vi "Hardware-HHCmdCalPoints.vi"(0 "HH Setup In":T1[](array[typedef]) {"Skip Fire Index" max=7; "Angles"."Duration [s]" format="%#_3p"; "Frequency [Hz]" format="%#_3p"}) -> (4 "HH Setup Out":T1[](array[typedef])=[{"Mode"=enum."Off", "Digital Input"=enum."Unused", "Polarity"=FALSE, "Frequency [Hz]"=0.0, "Duty Cycle [%]"=0.0, "TDC Offset [CAD]"=0.0, "Window Start [DBTDC]"=0.0, "Window End [DBTDC]"=0.0, "Angles"=[{"Enable"=FALSE, "Location [DBTDC]"=0.0, "Duration [s]"=0.0}, {"Enable"=FALSE, "Location [DBTDC]"=0.0, "Duration [s]"=0.0}, {"Enable"=FALSE, "Location [DBTDC]"=0.0, "Duration [s]"=0.0}, {"Enable"=FALSE, "Location [DBTDC]"=0.0, "Duration [s]"=0.0}], "Skip Fire"=FALSE, "Skip Fire Index"=0}, {"Mode"=enum."Off", "Digital Input"=enum."Unused", "Polarity"=FALSE, "Frequency [Hz]"=0.0, "Duty Cycle [%]"=0.0, "TDC Offset [CAD]"=0.0, "Window Start [DBTDC]"=0.0, "Window End [DBTDC]"=0.0, "Angles"=[{"Enable"=FALSE, "Location [DBTDC]"=0.0, "Duration [s]"=0.0}, {"Enable"=FALSE, "Location [DBTDC]"=0.0, "Duration [s]"=0.0}, {"Enable"=FALSE, "Location [DBTDC]"=0.0, "Duration [s]"=0.0}, {"Enable"=FALSE, "Location [DBTDC]"=0.0, "Duration [s]"=0.0}], "Skip Fire"=FALSE, "Skip Fire Index"=0}, {"Mode"=enum."Off", "Digital Input"=enum."Unused", "Polarity"=FALSE, "Frequency [Hz]"=0.0, "Duty Cycle [%]"=0.0, "TDC Offset [CAD]"=0.0, "Window Start [DBTDC]"=0.0, "Window End [DBTDC]"=0.0, "Angles"=[{"Enable"=FALSE, "Location [DBTDC]"=0.0, "Duration [s]"=0.0}, {"Enable"=FALSE, "Location [DBTDC]"=0.0, "Duration [s]"=0.0}, {"Enable"=FALSE, "Location [DBTDC]"=0.0, "Duration [s]"=0.0}, {"Enable"=FALSE, "Location [DBTDC]"=0.0, "Duration [s]"=0.0}], "Skip Fire"=FALSE, "Skip Fire Index"=0}, {"Mode"=enum."Off", "Digital Input"=enum."Unused", "Polarity"=FALSE, "Frequency [Hz]"=0.0, "Duty Cycle [%]"=0.0, "TDC Offset [CAD]"=0.0, "Window Start [DBTDC]"=0.0, "Window End [DBTDC]"=0.0, "Angles"=[{"Enable"=FALSE, "Location [DBTDC]"=0.0, "Duration [s]"=0.0}, {"Enable"=FALSE, "Location [DBTDC]"=0.0, "Duration [s]"=0.0}, {"Enable"=FALSE, "Location [DBTDC]"=0.0, "Duration [s]"=0.0}, {"Enable"=FALSE, "Location [DBTDC]"=0.0, "Duration [s]"=0.0}], "Skip Fire"=FALSE, "Skip Fire Index"=0}, {"Mode"=enum."Off", "Digital Input"=enum."Unused", "Polarity"=FALSE, "Frequency [Hz]"=0.0, "Duty Cycle [%]"=0.0, "TDC Offset [CAD]"=0.0, "Window Start [DBTDC]"=0.0, "Window End [DBTDC]"=0.0, "Angles"=[{"Enable"=FALSE, "Location [DBTDC]"=0.0, "Duration [s]"=0.0}, {"Enable"=FALSE, "Location [DBTDC]"=0.0, "Duration [s]"=0.0}, {"Enable"=FALSE, "Location [DBTDC]"=0.0, "Duration [s]"=0.0}, {"Enable"=FALSE, "Location [DBTDC]"=0.0, "Duration [s]"=0.0}], "Skip Fire"=FALSE, "Skip Fire Index"=0}, {"Mode"=enum."Off", "Digital Input"=enum."Unused", "Polarity"=FALSE, "Frequency [Hz]"=0.0, "Duty Cycle [%]"=0.0, "TDC Offset [CAD]"=0.0, "Window Start [DBTDC]"=0.0, "Window End [DBTDC]"=0.0, "Angles"=[{"Enable"=FALSE, "Location [DBTDC]"=0.0, "Duration [s]"=0.0}, {"Enable"=FALSE, "Location [DBTDC]"=0.0, "Duration [s]"=0.0}, {"Enable"=FALSE, "Location [DBTDC]"=0.0, "Duration [s]"=0.0}, {"Enable"=FALSE, "Location [DBTDC]"=0.0, "Duration [s]"=0.0}], "Skip Fire"=FALSE, "Skip Fire Index"=0}, {"Mode"=enum."Off", "Digital Input"=enum."Unused", "Polarity"=FALSE, "Frequency [Hz]"=0.0, "Duty Cycle [%]"=0.0, "TDC Offset [CAD]"=0.0, "Window Start [DBTDC]"=0.0, "Window End [DBTDC]"=0.0, "Angles"=[{"Enable"=FALSE, "Location [DBTDC]"=0.0, "Duration [s]"=0.0}, {"Enable"=FALSE, "Location [DBTDC]"=0.0, "Duration [s]"=0.0}, {"Enable"=FALSE, "Location [DBTDC]"=0.0, "Duration [s]"=0.0}, {"Enable"=FALSE, "Location [DBTDC]"=0.0, "Duration [s]"=0.0}], "Skip Fire"=FALSE, "Skip Fire Index"=0}, {"Mode"=enum."Off", "Digital Input"=enum."Unused", "Polarity"=FALSE, "Frequency [Hz]"=0.0, "Duty Cycle [%]"=0.0, "TDC Offset [CAD]"=0.0, "Window Start [DBTDC]"=0.0, "Window End [DBTDC]"=0.0, "Angles"=[{"Enable"=FALSE, "Location [DBTDC]"=0.0, "Duration [s]"=0.0}, {"Enable"=FALSE, "Location [DBTDC]"=0.0, "Duration [s]"=0.0}, {"Enable"=FALSE, "Location [DBTDC]"=0.0, "Duration [s]"=0.0}, {"Enable"=FALSE, "Location [DBTDC]"=0.0, "Duration [s]"=0.0}], "Skip Fire"=FALSE, "Skip Fire Index"=0}, {"Mode"=enum."Off", "Digital Input"=enum."Unused", "Polarity"=FALSE, "Frequency [Hz]"=0.0, "Duty Cycle [%]"=0.0, "TDC Offset [CAD]"=0.0, "Window Start [DBTDC]"=0.0, "Window End [DBTDC]"=0.0, "Angles"=[{"Enable"=FALSE, "Location [DBTDC]"=0.0, "Duration [s]"=0.0}, {"Enable"=FALSE, "Location [DBTDC]"=0.0, "Duration [s]"=0.0}, {"Enable"=FALSE, "Location [DBTDC]"=0.0, "Duration [s]"=0.0}, {"Enable"=FALSE, "Location [DBTDC]"=0.0, "Duration [s]"=0.0}], "Skip Fire"=FALSE, "Skip Fire Index"=0}, {"Mode"=enum."Off", "Digital Input"=enum."Unused", "Polarity"=FALSE, "Frequency [Hz]"=0.0, "Duty Cycle [%]"=0.0, "TDC Offset [CAD]"=0.0, "Window Start [DBTDC]"=0.0, "Window End [DBTDC]"=0.0, "Angles"=[{"Enable"=FALSE, "Location [DBTDC]"=0.0, "Duration [s]"=0.0}, {"Enable"=FALSE, "Location [DBTDC]"=0.0, "Duration [s]"=0.0}, {"Enable"=FALSE, "Location [DBTDC]"=0.0, "Duration [s]"=0.0}, {"Enable"=FALSE, "Location [DBTDC]"=0.0, "Duration [s]"=0.0}], "Skip Fire"=FALSE, "Skip Fire Index"=0}, {"Mode"=enum."Off", "Digital Input"=enum."Unused", "Polarity"=FALSE, "Frequency [Hz]"=0.0, "Duty Cycle [%]"=0.0, "TDC Offset [CAD]"=0.0, "Window Start [DBTDC]"=0.0, "Window End [DBTDC]"=0.0, "Angles"=[{"Enable"=FALSE, "Location [DBTDC]"=0.0, "Duration [s]"=0.0}, {"Enable"=FALSE, "Location [DBTDC]"=0.0, "Duration [s]"=0.0}, {"Enable"=FALSE, "Location [DBTDC]"=0.0, "Duration [s]"=0.0}, {"Enable"=FALSE, "Location [DBTDC]"=0.0, "Duration [s]"=0.0}], "Skip Fire"=FALSE, "Skip Fire Index"=0}, {"Mode"=enum."Off", "Digital Input"=enum."Unused", "Polarity"=FALSE, "Frequency [Hz]"=0.0, "Duty Cycle [%]"=0.0, "TDC Offset [CAD]"=0.0, "Window Start [DBTDC]"=0.0, "Window End [DBTDC]"=0.0, "Angles"=[{"Enable"=FALSE, "Location [DBTDC]"=0.0, "Duration [s]"=0.0}, {"Enable"=FALSE, "Location [DBTDC]"=0.0, "Duration [s]"=0.0}, {"Enable"=FALSE, "Location [DBTDC]"=0.0, "Duration [s]"=0.0}, {"Enable"=FALSE, "Location [DBTDC]"=0.0, "Duration [s]"=0.0}], "Skip Fire"=FALSE, "Skip Fire Index"=0}] {"Skip Fire Index" max=7; "Angles"."Duration [s]" format="%#_3p"; "Frequency [Hz]" format="%#_3p"})   [LabVIEW 2016, in "DSI-RT.lvlib"]
uses:
  DSI-RT.lvlib
  <vilib>/Powertrain Controls/Device Drivers/DCM/HH/RT/Setup.ctl
  <vilib>/Powertrain Controls/Device Drivers/DCM/HH/FPGA/Mode.ctl
  <vilib>/Powertrain Controls/Device Drivers/DCM/Rev0/FPGA/Digital Channel.ctl
  <vilib>/Powertrain Controls/Device Drivers/DCM/HH/RT/Angle Control.ctl
  <vilib>/addons/Software Calibration Management/xSCM/CalPoint.xnode
  <vilib>/addons/Software Calibration Management/xSCM/ni_scm.dll
  <vilib>/Powertrain Controls/Device Drivers/DCM/HH/RT/DCM - RT - HH.lvlib
  <vilib>/Powertrain Controls/Device Drivers/DCM/HH/FPGA/DCM - FPGA - HH.lvlib
  <vilib>/Powertrain Controls/Device Drivers/DCM/Rev0/FPGA/DCM - FPGA.lvlib
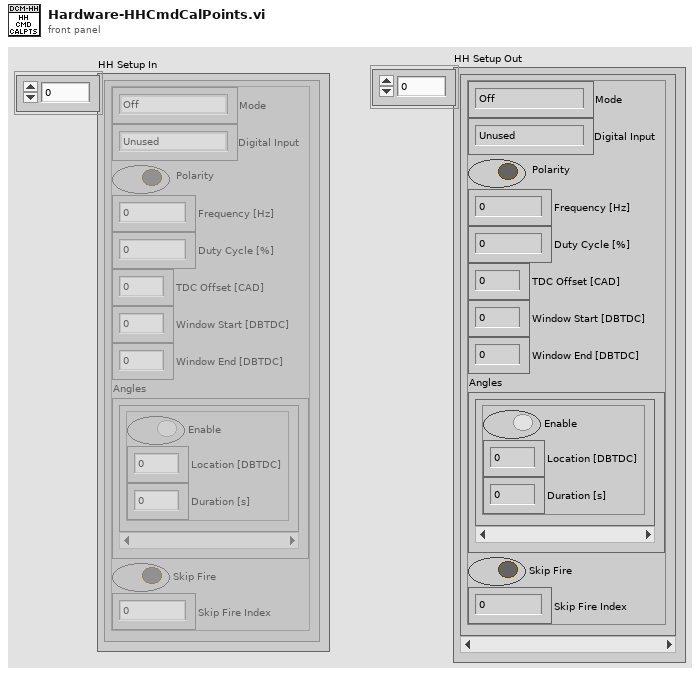
[diagram p1: front panel]
types:
  T1 = typedef "DCM - RT - HH.lvlib/Setup.ctl" = cluster{"Mode":T2, "Digital Input":T3, "Polarity":bool, "Frequency [Hz]":sgl, "Duty Cycle [%]":sgl, "TDC Offset [CAD]":sgl, "Window Start [DBTDC]":sgl, "Window End [DBTDC]":sgl, "Angles":T4[], "Skip Fire":bool, "Skip Fire Index":u8}
  T2 = typedef "DCM - FPGA - HH.lvlib/Mode.ctl" = enum8{"Off", "Direct", "Pulse Width Modulation", "Engine Position Tracking"}
  T3 = typedef "DCM - FPGA.lvlib/Digital Channel.ctl" = enum8{"Unused", "User OS", "Diff IO 1", "Diff IO 2", "Diff IO 3", "Diff IO 4", "Diff IO 5", "Diff IO 6", "Diff IO 7", "Diff IO 8", "Aux 1", "Aux 2", "Aux 3", "Aux 4", "Aux 5", "Aux 6", "Aux 7", "Aux 8", "Aux 9", "Aux 10", "Aux 11", "Aux 12", "Aux 13", "Aux 14", "Aux 15", "Aux 16"}
  T4 = typedef "DCM - RT - HH.lvlib/Angle Control.ctl" = cluster{"Enable":bool, "Location [DBTDC]":sgl, "Duration [s]":sgl}
  T5 = cluster{"Mode":enum8{"Off", "Direct", "Pulse Width Modulation", "Engine Position Tracking"}, "Digital Input":enum8{"Unused", "User OS", "Diff IO 1", "Diff IO 2", "Diff IO 3", "Diff IO 4", "Diff IO 5", "Diff IO 6", "Diff IO 7", "Diff IO 8", "Aux 1", "Aux 2", "Aux 3", "Aux 4", "Aux 5", "Aux 6", "Aux 7", "Aux 8", "Aux 9", "Aux 10", "Aux 11", "Aux 12", "Aux 13", "Aux 14", "Aux 15", "Aux 16"}, "Polarity":bool, "Frequency [Hz]":sgl, "Duty Cycle [%]":sgl, "TDC Offset [CAD]":sgl, "Window Start [DBTDC]":sgl, "Window End [DBTDC]":sgl, "Angles":cluster{"Enable":bool, "Location [DBTDC]":sgl, "Duration [s]":sgl}[], "Skip Fire":bool, "Skip Fire Index":u8}[]
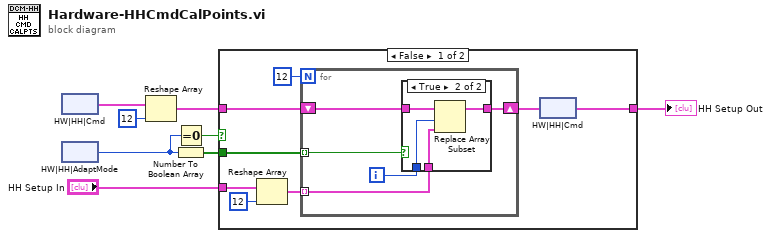
[diagram p0: block diagram]
diagram:
  n1 = xnode "HW|HH|Cmd"() -> ("Value"=w3:T5)
  n2 = xnode "HW|HH|AdaptMode"() -> ("Value"=w1:u32)
  n3 = Reshape Array(w3, 12 ("dimension size")) -> (w8:T5)
  n4 = Equal To 0?(x=w1) -> (x = 0?=w5:bool)
  n5 = Number To Boolean Array(number=w1) -> (Boolean array=w6:bool[])
  n6 = case shown="False" w5 {
    tunnel: w8 -> [w15 w31]
    tunnel: [w9 w31] -> w4
    tunnel: w6 -> [w13 _]
    tunnel: "HH Setup In" -> [w10 _]
    frame False {
      n7 = Reshape Array(w10, 12 ("dimension size")) -> (w11:T1[])
      n8 = for {
        N: 12 -> [_]
        tunnel: w13 -> [w22] mode=indexing
        shift-right: [w24] -> w9
        shift-left: w15 -> [w25]
        tunnel: w11 -> [w21] mode=indexing
        i -> [w23]
        n9 = case shown="True" w22 {
          tunnel: w25 -> [w26 w30]
          tunnel: [w26 w29] -> w24
          tunnel: w23 -> [_ w28]
          tunnel: w21 -> [_ w27]
          frame False {
          }
          frame True {
            n10 = Replace Array Subset(array=w30, new element=w27, index=w28) -> (w29:T5)
          }
        }
      }
      n11 = xnode "HW|HH|Cmd"("Value"=w9) -> ()
    }
    frame True {
    }
  }
  "HH Setup Out" <- w4
